vi "Setup_instrument.vi"(8 "error in (no error)":errorcluster, 10 "Y-Axis Visa Resource Name":refnum<visa-resource-name>, 11 "Z-Axis Visa Resource Name":refnum<visa-resource-name>) -> (0 "error out":errorcluster, 2 "Y-Axis Visa Resource Name (out)":refnum<visa-resource-name>, 3 "Z-Axis Visa Resource Name (out)":refnum<visa-resource-name>)   [LabVIEW 2019]
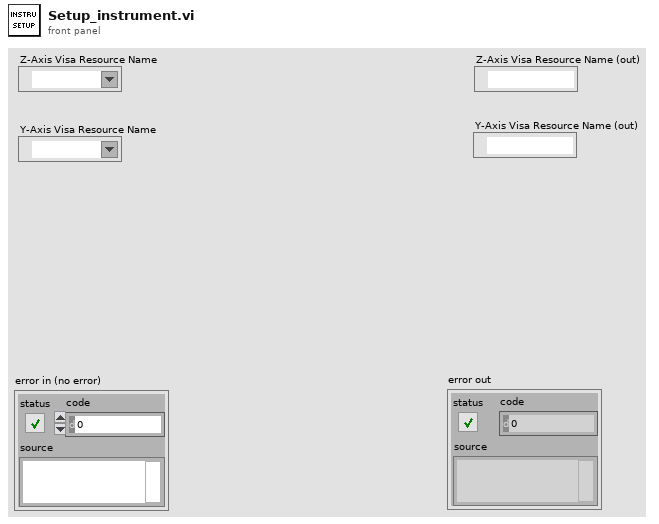
[diagram p1: front panel]
types:
  T1 = cluster{"Max Current Z-Axis (A)":dbl, "Max Ramp Rate Z-Axis (A/s)":dbl, "Coil Constant Z-Axis (T/A)":dbl, "Inductance Z-Axis (H)":dbl, "Switch Heater Current Z-Axis (mA)":dbl, "Max Current Y-Axis (A)":dbl, "Max Ramp Rate Y-Axis (A/s)":dbl, "Coil Constant Y-Axis (T/A)":dbl, "Inductance Y-Axis (H)":dbl, "Switch Heater Current Y-Axis (mA)":dbl, "Switch Heater Z-Axis Installed?":bool, "Switch Heater Y-Axis Installed?":bool, "Field Units":u16, "Ramp Units":u16, "Z-Axis Switch Heater Cooling Time":dbl, "Z-Axis Switch Heater Heating Time":dbl, "Y-Axis Switch Heater Cooling Time":dbl, "Y-Axis Switch Heater Heating Time":dbl}
  T2 = cluster{"error":bool, "code":i32, "source":string}
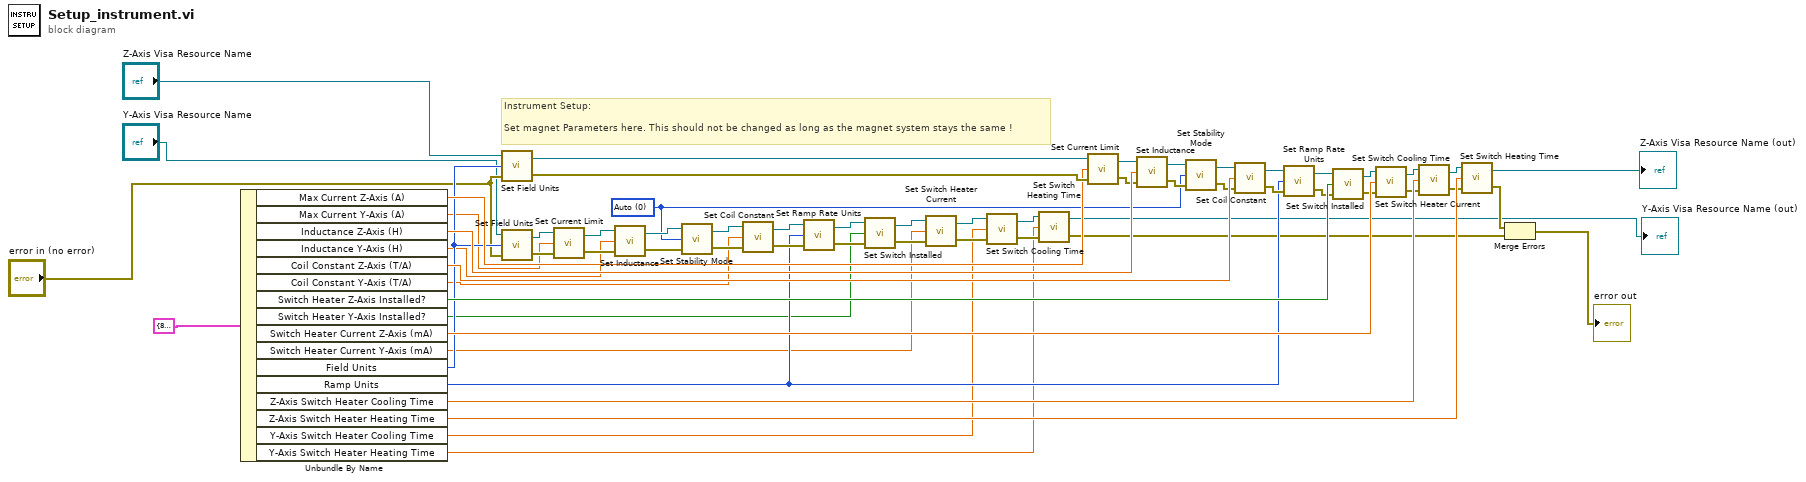
[diagram p0: block diagram]
diagram:
  w16 = u16 0 items=["Auto", "Manual", "Test"] ("Stability Mode")
  # "Instrument Setup:\n\nSet magnet Parameters here. This should not be changed as long as the magnet system stays the same !"
  n1 = Unbundle By Name(T1 {"Max Current Z-Axis (A)"=84.51, "Max Ramp Rate Z-Axis (A/s)"=0.203, "Coil Constant Z-Axis (T/A)"=0.1065, "Inductance Z-Axis (H)"=9.9, "Switch Heater Current Z-Axis (mA)"=49.0, "Max Current Y-Axis (A)"=98.91, "Max Ramp Rate Y-Axis (A/s)"=0.065, "Coil Constant Y-Axis (T/A)"=0.0455, "Inductance Y-Axis (H)"=30.7, "Switch Heater Current Y-Axis (mA)"=56.0, "Switch Heater Z-Axis Installed?"=TRUE, "Switch Heater Y-Axis Installed?"=TRUE, "Field Units"=1, "Ramp Units"=1, "Z-Axis Switch Heater Cooling Time"=20.0, "Z-Axis Switch Heater Heating Time"=20.0, "Y-Axis Switch Heater Cooling Time"=20.0, "Y-Axis Switch Heater Heating Time"=20.0} ("AMI_Parameters")) -> ("Max Current Z-Axis (A)"=w56:dbl, "Max Current Y-Axis (A)"=w18:dbl, "Inductance Z-Axis (H)"=w55:dbl, "Inductance Y-Axis (H)"=w17:dbl, "Coil Constant Z-Axis (T/A)"=w54:dbl, "Coil Constant Y-Axis (T/A)"=w15:dbl, "Switch Heater Z-Axis Installed?"=w52:bool, "Switch Heater Y-Axis Installed?"=w13:bool, "Switch Heater Current Z-Axis (mA)"=w51:dbl, "Switch Heater Current Y-Axis (mA)"=w12:dbl, "Field Units"=w19:u16, "Ramp Units"=w14:u16, "Z-Axis Switch Heater Cooling Time"=w49:dbl, "Z-Axis Switch Heater Heating Time"=w40:dbl, "Y-Axis Switch Heater Cooling Time"=w11:dbl, "Y-Axis Switch Heater Heating Time"=w10:dbl)
  n2 = call "Set Field Units.vi"("error in"="error in (no error)", "Field Units"=w19, "VISA resource name"="Z-Axis Visa Resource Name") -> ("error out"=w60:T2, "VISA resource name out"=w62:refnum<visa-resource-name>)
  n3 = call "Set Field Units.vi"("error in"="error in (no error)", "Field Units"=w19, "VISA resource name"="Y-Axis Visa Resource Name") -> ("error out"=w35:T2, "VISA resource name out"=w37:refnum<visa-resource-name>)
  n4 = call "Set Current Limit.vi"("error in"=w35, "Current Limit (A)"=w18, "VISA resource name"=w37) -> ("error out"=w27:T2, "VISA resource name out"=w28:refnum<visa-resource-name>)
  n5 = call "Set Inductance.vi"("error in"=w27, "Magnet Inductance (H)"=w17, "connection ID"=w28) -> ("error out"=w34:T2, "connection ID out"=w36:refnum<visa-resource-name>)
  n6 = call "Set Stability Mode.vi"("error in"=w34, "Stability Mode"=w16, "connection ID"=w36) -> ("error out"=w26:T2, "connection ID out"=w25:refnum<visa-resource-name>)
  n7 = call "Set Coil Constant.vi"("error in"=w26, "Coil Constant (kG/A)"=w15, "VISA resource name"=w25) -> ("error out"=w33:T2, "VISA resource name out"=w32:refnum<visa-resource-name>)
  n8 = call "Set Ramp Rate Units.vi"("error in"=w33, "Ramp Rate Units"=w14, "VISA resource name"=w32) -> ("error out"=w30:T2, "VISA resource name out"=w31:refnum<visa-resource-name>)
  n9 = call "Set Switch Installed.vi"("error in"=w30, "Switch is Installed"=w13, "VISA resource name"=w31) -> ("error out"=w23:T2, "VISA resource name out"=w22:refnum<visa-resource-name>)
  n10 = call "Set Switch Heater Current.vi"("error in"=w23, "Switch Heater Current (mA)"=w12, "VISA resource name"=w22) -> ("error out"=w24:T2, "VISA resource name out"=w29:refnum<visa-resource-name>)
  n11 = call "Set Switch Cooling Time.vi"("error in"=w24, "Switch Cooling Time (sec)"=w11, "connection ID"=w29) -> ("error out"=w21:T2, "connection ID out"=w20:refnum<visa-resource-name>)
  n12 = call "Set Switch Heating Time.vi"("error in"=w21, "Switch Heating Time (sec)"=w10, "VISA resource name"=w20) -> ("error out"=w9:T2, "VISA resource name out"=→"Y-Axis Visa Resource Name (out)":refnum<visa-resource-name>)
  n13 = call "Set Current Limit.vi"("error in"=w60, "Current Limit (A)"=w56, "VISA resource name"=w62) -> ("error out"=w46:T2, "VISA resource name out"=w47:refnum<visa-resource-name>)
  n14 = call "Set Inductance.vi"("error in"=w46, "Magnet Inductance (H)"=w55, "connection ID"=w47) -> ("error out"=w59:T2, "connection ID out"=w61:refnum<visa-resource-name>)
  n15 = call "Set Stability Mode.vi"("error in"=w59, "Stability Mode"=w16, "connection ID"=w61) -> ("error out"=w45:T2, "connection ID out"=w44:refnum<visa-resource-name>)
  n16 = call "Set Coil Constant.vi"("error in"=w45, "Coil Constant (kG/A)"=w54, "VISA resource name"=w44) -> ("error out"=w58:T2, "VISA resource name out"=w57:refnum<visa-resource-name>)
  n17 = call "Set Ramp Rate Units.vi"("error in"=w58, "Ramp Rate Units"=w14, "VISA resource name"=w57) -> ("error out"=w50:T2, "VISA resource name out"=w53:refnum<visa-resource-name>)
  n18 = call "Set Switch Installed.vi"("error in"=w50, "Switch is Installed"=w52, "VISA resource name"=w53) -> ("error out"=w42:T2, "VISA resource name out"=w41:refnum<visa-resource-name>)
  n19 = call "Set Switch Heater Current.vi"("error in"=w42, "Switch Heater Current (mA)"=w51, "VISA resource name"=w41) -> ("error out"=w43:T2, "VISA resource name out"=w48:refnum<visa-resource-name>)
  n20 = call "Set Switch Cooling Time.vi"("error in"=w43, "Switch Cooling Time (sec)"=w49, "connection ID"=w48) -> ("error out"=w39:T2, "connection ID out"=w38:refnum<visa-resource-name>)
  n21 = call "Set Switch Heating Time.vi"("error in"=w39, "Switch Heating Time (sec)"=w40, "VISA resource name"=w38) -> ("error out"=w8:T2, "VISA resource name out"=→"Z-Axis Visa Resource Name (out)":refnum<visa-resource-name>)
  n22 = Merge Errors(w8, w9) -> (→"error out":errorcluster)
